vi "Serial test.vi"() -> ()   [LabVIEW 2016]
panel:
  out "read buffer":string
  in  "Exit":bool
  in  "Send data":bool
  in  "Value":sgl min=0 max=204.8 step=0.0125 format="%#_g V"
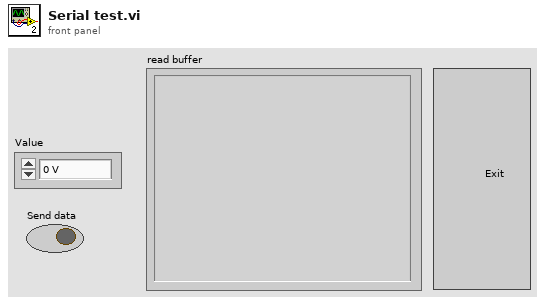
[diagram p1: front panel]
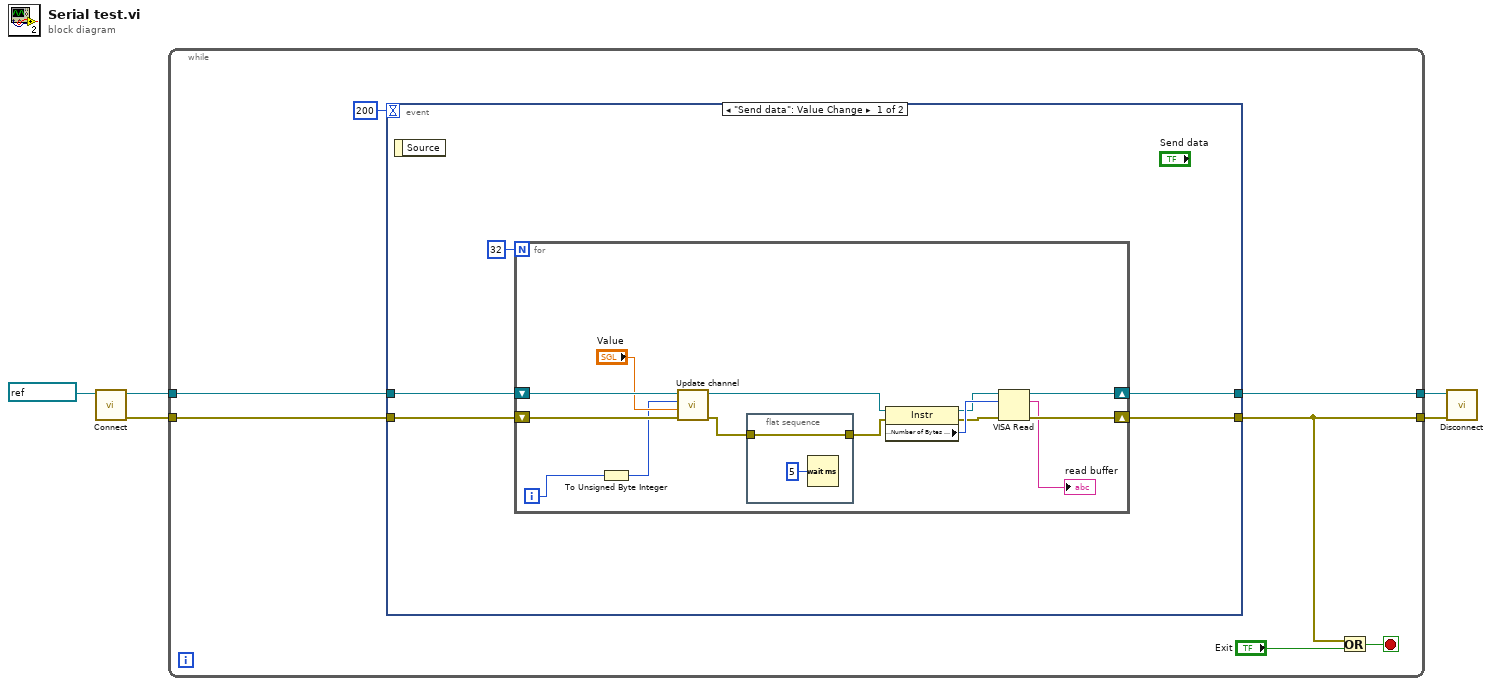
[diagram p0: block diagram]
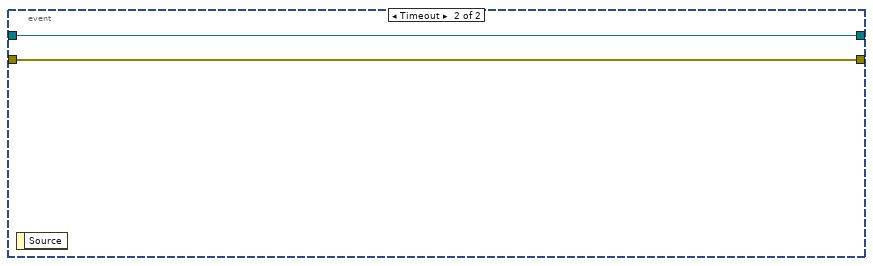
[diagram p2: hidden frame]
diagram:
  n1 = call "Connect.vi"("Arduino Port"=refnum<visa-resource-name> "COM14") -> ("Error Out"=w4:errorcluster, "Arduino Port out"=w5:refnum<visa-resource-name>)  [unwired: 9 in]
  n2 = while {
    tunnel: w5 -> [w12]
    tunnel: w4 -> [w11]
    tunnel: [w10] -> w3
    tunnel: [w7] -> w2
    stop <- w9 stop-if-true
    n3 = event shown="[0] \"Send data\": Value Change" {
      selector: _ -> [_ _]
      dyn-events: _ -> [_ _]
      timeout: 200 -> [_ _]
      tunnel: w12 -> [w17 w35]
      tunnel: w11 -> [w16 w34]
      tunnel: [w15 w35] -> w10
      tunnel: [w14 w34] -> w7
      event "Send data": Value Change {
        n4 = event-data() -> ()  [unwired: 1 in, 1 out]
        n5 = for {
          N: 32 -> [_]
          shift-right: [w29] -> w15
          shift-left: w17 -> [w31]
          shift-right: [w28] -> w14
          shift-left: w16 -> [w30]
          i -> [w19]
          n6 = To Unsigned Byte Integer(number=w19) -> (unsigned 8bit integer=w18:u8)
          n7 = call "Update channel.vi"("Error In"=w30, "Value"="Value", "Channel"=w18, "Arduino Port"=w31) -> ("Error Out"=w21:errorcluster, "Arduino Port out"=w27:refnum<visa-resource-name>)  [unwired: 6 in]
          n8 = flat-sequence {
            tunnel: w21 -> [w33]
            tunnel: [w33] -> w20
            frame #0 {
              n9 = Wait (ms)(milliseconds to wait=u32 5) -> ()  [unwired: 1 out]
            }
          }
          n10 = property class="Instr"(reference=w27, error in=w20) -> (reference out=w24:refnum<visa-resource-name>, error out=w25:errorcluster, "Serial Settings:Number of Bytes at Serial Port"=w26:u32)
          n11 = VISA Read(VISA resource name=w24, byte count=w26, error in (no error)=w25) -> (VISA resource name out=w29:refnum<visa-resource-name>, read buffer=→"read buffer":string, error out=w28:errorcluster)  [unwired: 1 out]
        }
      }
      event Timeout {
        n12 = event-data() -> ()  [unwired: 1 in, 1 out]
      }
    }
    n13 = Or(x=w7, y="Exit") -> (x .or. y?=w9:bool)
  }
  n14 = call "Disconnect.vi"("Error In"=w2, "Arduino Port"=w3) -> ()  [unwired: 9 in, 1 out]
